vi "is_empty.vi"(8 "error in (no error)":errorcluster, 11 "ImageCollection in":refnum<class "ImageCollection.lvclass">) -> (0 "error out":errorcluster, 2 "is empty?":bool, 3 "ImageCollection out":refnum<class "ImageCollection.lvclass">)   [LabVIEW 2010, in "ImageCollection.lvclass"]
uses:
  ImageCollection.lvclass
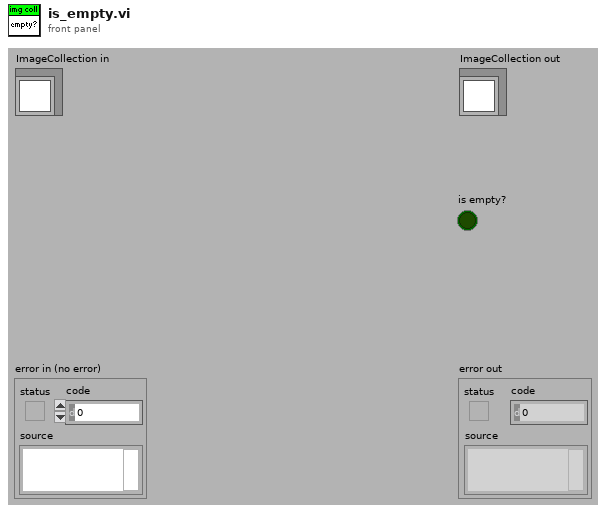
[diagram p1: front panel]
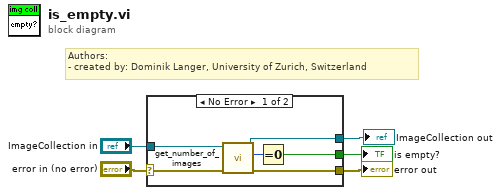
[diagram p0: block diagram]
diagram:
  # "Authors: \n- created by: Dominik Langer, University of Zurich, Switzerland"
  n1 = case shown="No Error" "error in (no error)" {
    selector: "error in (no error)" -> [w7 w13]
    tunnel: [w6 w13] -> w4
    tunnel: [w8 w12] -> w2
    tunnel: "ImageCollection in" -> [w9 w12]
    tunnel: [w10 _] -> w1
    frame No Error {
      n2 = call-dynamic "get_number_of_images.vi"("error in (no error)"=w7, "ImageCollection in"=w9) -> ("error out"=w6:errorcluster, "size"=w11:i32, "ImageCollection out"=w8:refnum<class "ImageCollection.lvclass">)  [unwired: 7 out]
      n3 = Equal To 0?(x=w11) -> (x = 0?=w10:bool)
    }
    frame Error {
    }
  }
  "error out" <- w4
  "ImageCollection out" <- w2
  "is empty?" <- w1
